vi "LINC Read Command.vi"(8 "error in (no error)":errorcluster, 9 "Options":T1, 10 "start field (default)":i32=-1, 11 "LINC session":refnum<class "LINC.lvclass">) -> (0 "error out":errorcluster, 1 "cmd data":string, 2 "cmd name":string, 3 "dup LINC session":refnum<class "LINC.lvclass">, 4 "application command":bool, 5 "GUID":string, 6 "cmd text":string, 7 "cmd origin":T2)   [LabVIEW 2018, in "STEPkgDriver_LINC.lvlib" / "LINC.lvclass"]
uses:
  LINC.lvclass
  STEPkgDriver_LINC.lvlib
  LINC Global Mode.ctl
  LINC Command Origin.ctl
  LINC Read Command Options.ctl
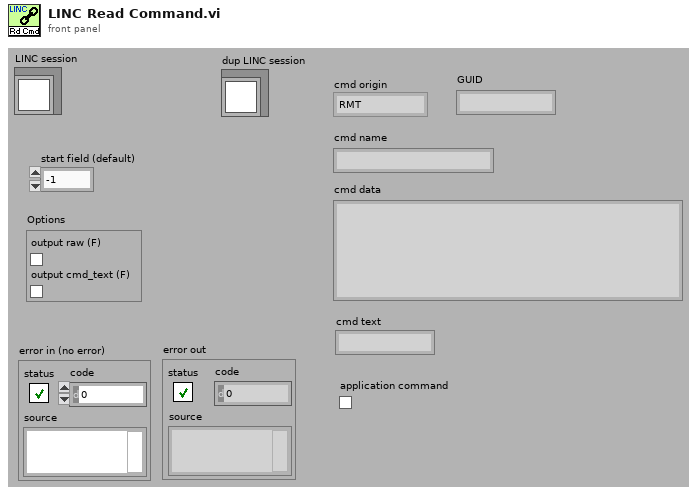
[diagram p1: front panel]
types:
  T1 = typedef "STEPkgDriver_LINC.lvlib/LINC Read Command Options.ctl" = cluster{"output raw (F)":bool, "output cmd_text (F)":bool}
  T2 = typedef "STEPkgDriver_LINC.lvlib/LINC Command Origin.ctl" = enum8{"RMT", "LCL"}
  T3 = typedef "STEPkgDriver_LINC.lvlib/LINC Global Mode.ctl" = enum16{"INIT", "CLEAR", "ADD_PKT_HDR", "ADD_PKT", "GET_PKT_NAMES", "GET_PKT_DESC", "GET_PKT_HDR", "GET_PKT", "SET_PKT", "SET_DATA", "SIM_EN", "SIM_DS"}
  T4 = typedef "STEPkgDriver_LINC.lvlib/LINC Format Prototype.ctl" = cluster{"type":string, "bit offset":i32, "bit size":i32, "format":string, "unit":string, "description":string, "state values":i64[], "states":string[], "max":string, "min":string, "default":string, "array":bool, "bit element size":i32, "poly bound":dbl[], "poly scale":cluster{"coefficients":dbl[]}[], "labview size":i32, "simulate":bool, "ID":bool, "required":bool}
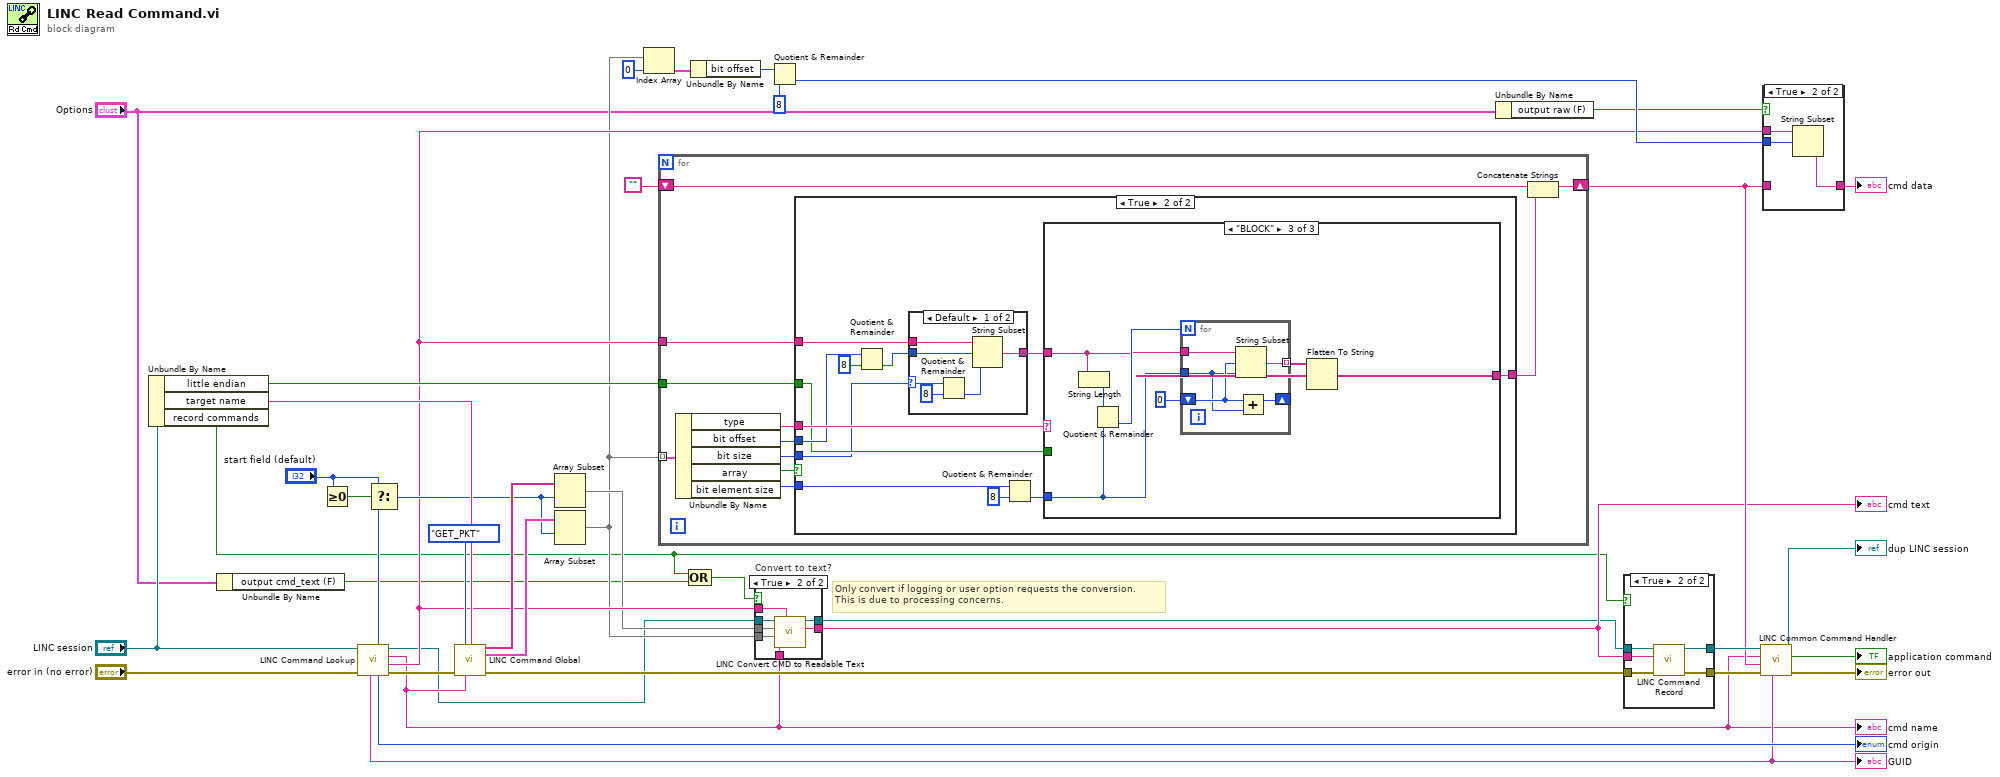
[diagram p0: block diagram]
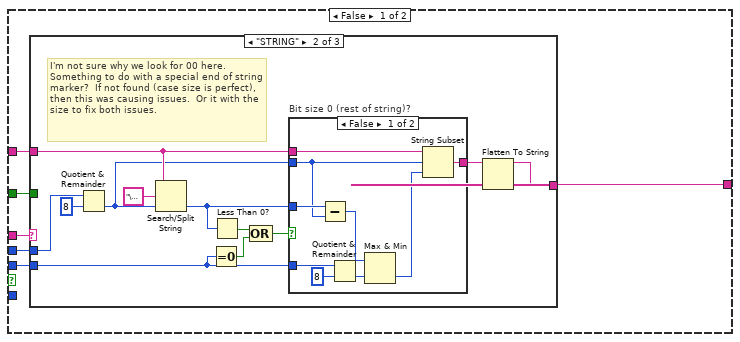
[diagram p3: hidden frame]
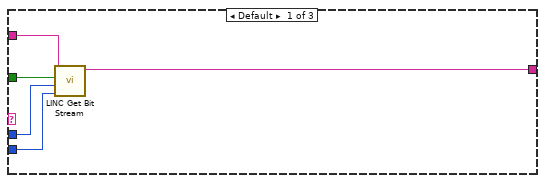
[diagram p4: hidden frame]
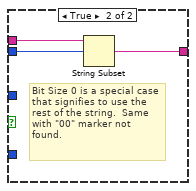
[diagram p5: hidden frame]
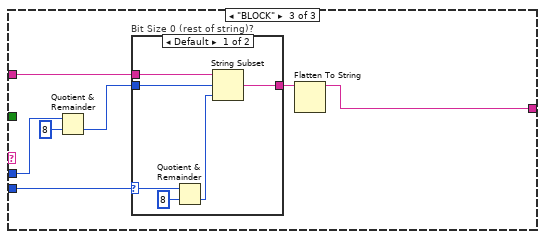
[diagram p6: hidden frame]
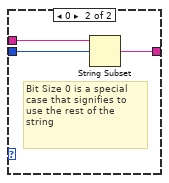
[diagram p7: hidden frame]
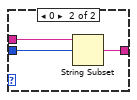
[diagram p8: hidden frame]
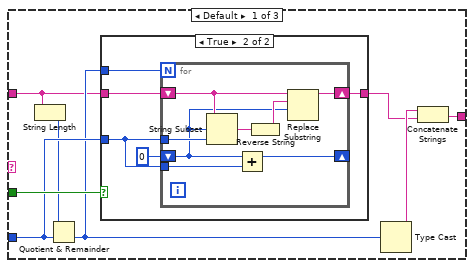
[diagram p9: hidden frame]
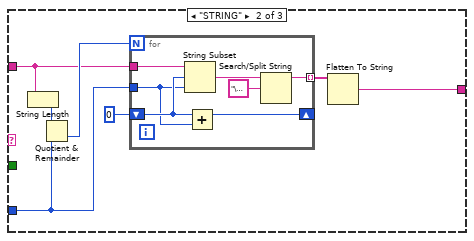
[diagram p11: hidden frame]
diagram:
  # "Only convert if logging or user option requests the conversion.\nThis is due to processing concerns."
  n1 = Unbundle By Name("LINC session") -> ("little endian"=w29:bool, "target name"=w32:string, "record commands"=w3:bool)
  n2 = Unbundle By Name("Options") -> ("output cmd_text (F)"=w2:bool)
  n3 = Greater Or Equal To 0?(x="start field (default)") -> (x >= 0?=w28:bool)
  n4 = call "LINC Command Lookup.vi"("error in (no error)"="error in (no error)", "LINC session"="LINC session") -> ("error out"=w31:errorcluster, "cmd data"=w13:string, "cmd name"=w12:string, "dup LINC session"=w8:refnum<class "LINC.lvclass">, "cmd origin"=→"cmd origin":T2, "cmd header fields"=w27:i32, "cmd GUID"=w14:string)  [unwired: 3 in]
  "cmd name" <- w12
  "GUID" <- w14
  n5 = Select(t="start field (default)", s=w28, f=w27) -> (s? t:f=w16:i32)
  n6 = call "LINC Command Global.vi"("mode"=LINC_Global_Mode."GET_PKT", "target name"=w32, "error in (no error)"=w31, "packet name"=w12) -> ("values out"=w18:string[], "item formats out"=w17:T4[], "error out"=w36:errorcluster)  [unwired: 7 in, 2 out]
  n7 = Array Subset(array=w18, index=w16) -> (w11:string[])  [unwired: 1 in]
  n8 = Array Subset(array=w17, index=w16) -> (w10:T4[])  [unwired: 1 in]
  n9 = Index Array(array=w10, index=0) -> (element=w23:T4)
  n10 = for {
    shift-right: [w51] -> w19
    shift-left: "" -> [w45]
    tunnel: w13 -> [w46]
    tunnel: w29 -> [w42]
    tunnel: w10 -> [w41] mode=indexing
    n11 = Unbundle By Name(w41) -> ("type"=w47:string, "bit offset"=w43:i32, "bit size"=w50:i32, "array"=w48:bool, "bit element size"=w49:i32)
    n12 = case shown="True" w48 {
      tunnel: w47 -> [w57 w113]
      tunnel: w50 -> [w55 w103]
      tunnel: [w56 w114] -> w44
      tunnel: w49 -> [_ w110]
      tunnel: w43 -> [w53 w106]
      tunnel: w46 -> [w54 w107]
      tunnel: w42 -> [w52 w104]
      frame False {
        n13 = case shown="\"STRING\"" w57 {
          tunnel: w55 -> [w60 w64 w87]
          tunnel: [w59 w69 w89] -> w56
          tunnel: w54 -> [w62 w71 w91]
          tunnel: w53 -> [w61 w72 w92]
          tunnel: w52 -> [w58 _ _]
          frame Default {
            n14 = call "LINC Get Bit Stream.vi"("bit size"=w60, "bit offset"=w61, "little endian"=w58, "data in"=w62) -> ("data out"=w59:string)  [unwired: 6 in, 1 out]
          }
          frame "STRING" {
            # "I'm not sure why we look for 00 here. Something to do with a special end of string marker?  If not found (case size is perfect), then this was causing issues.  Or it with the size to fix both issues."
            n15 = Quotient & Remainder(x=w72, y=8) -> (floor(x/y)=w70:i32)  [unwired: 1 out]
            n16 = Search/Split String(string=w71, search string/char (-)="\u0000", offset (0)=w70) -> (offset of match=w67:i32)  [unwired: 2 out]
            n17 = Equal To 0?(x=w64) -> (x = 0?=w65:bool)
            n18 = Less Than 0?(x=w67) -> (x < 0?=w66:bool)
            n19 = Compound Arithmetic op=OR(w66, w65) -> (w63:bool)
            n20 = case "Bit size 0 (rest of string)?" shown="False" w63 {
              tunnel: w71 -> [w83 w86]
              tunnel: w67 -> [w82 _]
              tunnel: w70 -> [w81 w85]
              tunnel: [w76 w84] -> w68
              tunnel: w64 -> [w75 _]
              frame False {
                n21 = Subtract(x=w82, y=w81) -> (x-y=w79:i32)
                n22 = Quotient & Remainder(x=w75, y=8) -> (floor(x/y)=w78:i32)  [unwired: 1 out]
                n23 = Max & Min(x=w79, y=w78) -> (min(x,y)=w77:i32)  [unwired: 1 out]
                n24 = String Subset(string=w83, offset (0)=w81, length (rest)=w77) -> (substring=w76:string)
              }
              frame True {
                # "Bit Size 0 is a special case that signifies to use the rest of the string.  Same with \"00\" marker not found."
                n25 = String Subset(string=w86, offset (0)=w85) -> (substring=w84:string)  [unwired: 1 in]
              }
            }
            n26 = Flatten To String(anything=w68) -> (data string=w69:string)  [unwired: 3 in, 2 out]
          }
          frame "BLOCK" {
            n27 = Quotient & Remainder(x=w92, y=8) -> (floor(x/y)=w90:i32)  [unwired: 1 out]
            n28 = case "Bit Size 0 (rest of string)?" shown="Default" w87 {
              selector: w87 -> [w94 _]
              tunnel: w91 -> [w99 w102]
              tunnel: w90 -> [w98 w100]
              tunnel: [w97 w101] -> w88
              frame Default {
                n29 = Quotient & Remainder(x=w94, y=8) -> (floor(x/y)=w96:i32)  [unwired: 1 out]
                n30 = String Subset(string=w99, offset (0)=w98, length (rest)=w96) -> (substring=w97:string)
              }
              frame 0 {
                # "Bit Size 0 is a special case that signifies to use the rest of the string"
                n31 = String Subset(string=w102, offset (0)=w100) -> (substring=w101:string)  [unwired: 1 in]
              }
            }
            n32 = Flatten To String(anything=w88) -> (data string=w89:string)  [unwired: 3 in, 2 out]
          }
        }
      }
      frame True {
        n33 = Quotient & Remainder(x=w106, y=8) -> (floor(x/y)=w109:i32)  [unwired: 1 out]
        n34 = case shown="Default" w103 {
          selector: w103 -> [w115 _]
          tunnel: w109 -> [w120 w123]
          tunnel: w107 -> [w118 w122]
          tunnel: [w117 w121] -> w105
          frame Default {
            n35 = Quotient & Remainder(x=w115, y=8) -> (floor(x/y)=w116:i32)  [unwired: 1 out]
            n36 = String Subset(string=w118, offset (0)=w120, length (rest)=w116) -> (substring=w117:string)
          }
          frame 0 {
            n37 = String Subset(string=w122, offset (0)=w123) -> (substring=w121:string)  [unwired: 1 in]
          }
        }
        n38 = Quotient & Remainder(x=w110, y=8) -> (floor(x/y)=w111:i32)  [unwired: 1 out]
        n39 = case shown="\"BLOCK\"" w113 {
          tunnel: [w130 w148 w162] -> w114
          tunnel: w111 -> [w127 w150 w164]
          tunnel: w105 -> [w125 w147 w161]
          tunnel: w104 -> [w128 _ _]
          frame Default {
            n40 = String Length(string=w125) -> (length=w124:i32)
            n41 = Quotient & Remainder(x=w124, y=w127) -> (floor(x/y)=w126:i32)  [unwired: 1 out]
            n42 = case shown="True" w128 {
              tunnel: w125 -> [w132 w136]
              tunnel: [w132 w135] -> w129
              tunnel: w127 -> [_ w134]
              tunnel: w126 -> [_ w133]
              frame False {
              }
              frame True {
                n43 = for {
                  N: w133 -> [_]
                  shift-right: [w140] -> w135
                  shift-left: w136 -> [w141]
                  shift-right: [w144] -> _
                  shift-left: 0 -> [w138]
                  tunnel: w134 -> [w145]
                  tunnel: w134 -> [w143]
                  n44 = String Subset(string=w141, offset (0)=w138, length (rest)=w145) -> (substring=w142:string)
                  n45 = Add(x=w138, y=w143) -> (x+y=w144:i32)
                  n46 = Reverse String(1:w142) -> (0:w139:string)
                  n47 = Replace Substring(3:w138, 4:w139, 5:w141) -> (1:w140:string)  [unwired: 1 in, 1 out]
                }
              }
            }
            n48 = Type Cast(x=w126) -> (*(type *) &x=w131:string)  [unwired: 1 in]
            n49 = Concatenate Strings(w131, w129) -> (w130:string)
          }
          frame "STRING" {
            n50 = String Length(string=w147) -> (length=w146:i32)
            n51 = Quotient & Remainder(x=w146, y=w150) -> (floor(x/y)=w151:i32)  [unwired: 1 out]
            n52 = for {
              N: w151 -> [_]
              tunnel: w150 -> [w156]
              tunnel: w147 -> [w159]
              shift-right: [w157] -> _
              shift-left: 0 -> [w158]
              tunnel: [w153] -> w149 mode=indexing
              n53 = String Subset(string=w159, offset (0)=w158, length (rest)=w156) -> (substring=w154:string)
              n54 = Add(x=w158, y=w156) -> (x+y=w157:i32)
              n55 = Search/Split String(string=w154, search string/char (-)="\u0000") -> (substring before match=w153:string)  [unwired: 3 out]
            }
            n56 = Flatten To String(anything=w149) -> (data string=w148:string)  [unwired: 3 in, 2 out]
          }
          frame "BLOCK" {
            n57 = String Length(string=w161) -> (length=w160:i32)
            n58 = Quotient & Remainder(x=w160, y=w164) -> (floor(x/y)=w165:i32)  [unwired: 1 out]
            n59 = for {
              N: w165 -> [_]
              tunnel: w164 -> [w168]
              tunnel: w161 -> [w171]
              shift-right: [w169] -> _
              shift-left: 0 -> [w170]
              tunnel: [w167] -> w163 mode=indexing
              n60 = String Subset(string=w171, offset (0)=w170, length (rest)=w168) -> (substring=w167:string)
              n61 = Add(x=w170, y=w168) -> (x+y=w169:i32)
            }
            n62 = Flatten To String(anything=w163) -> (data string=w162:string)  [unwired: 3 in, 2 out]
          }
        }
      }
    }
    n63 = Concatenate Strings(w45, w44) -> (w51:string)
  }
  n64 = Compound Arithmetic op=OR(w3, w2) -> (w1:bool)
  n65 = Unbundle By Name(w23) -> ("bit offset"=w22:i32)
  n66 = case "Convert to text?" shown="True" w1 {
    tunnel: w13 -> [_ w179]
    tunnel: w12 -> [_ w178]
    tunnel: w11 -> [_ w177]
    tunnel: w10 -> [_ w176]
    tunnel: [_ w175] -> w9
    tunnel: w8 -> [w172 w174]
    tunnel: [w172 w173] -> w6
    frame False {
    }
    frame True {
      n67 = call "LINC Convert CMD to Readable Text.vi"("command name in"=w178, "command data in"=w179, "parameter formats"=w176, "parameter names"=w177, "LINC in"=w174) -> ("Cmd Text"=w175:string, "LINC out"=w173:refnum<class "LINC.lvclass">)  [unwired: 5 in]
    }
  }
  "cmd text" <- w9
  n68 = Quotient & Remainder(x=w22, y=8) -> (floor(x/y)=w20:i32)  [unwired: 1 out]
  n69 = Unbundle By Name("Options") -> ("output raw (F)"=w5:bool)
  n70 = case shown="True" w3 {
    tunnel: [w180 w186] -> w37
    tunnel: w36 -> [w180 w185]
    tunnel: [w181 w184] -> w35
    tunnel: w6 -> [w181 w183]
    tunnel: w9 -> [_ w182]
    frame False {
    }
    frame True {
      n71 = call "LINC Command Record.vi"("error in (no error)"=w185, "command text"=w182, "LINC session"=w183) -> ("error out"=w186:errorcluster, "dup LINC session"=w184:refnum<class "LINC.lvclass">)  [unwired: 7 in]
    }
  }
  n72 = call "LINC Common Command Handler.vi"("GUID"=w14, "error in (no error)"=w37, "command data in"=w19, "command name in"=w12, "LINC session"=w35) -> ("error out"=→"error out":errorcluster, "application command"=→"application command":bool, "dup LINC session"=→"dup LINC session":refnum<class "LINC.lvclass">)  [unwired: 4 in]
  n73 = case shown="True" w5 {
    tunnel: w13 -> [_ w190]
    tunnel: [w187 w189] -> w24
    tunnel: w20 -> [_ w188]
    tunnel: w19 -> [w187 _]
    frame False {
    }
    frame True {
      n74 = String Subset(string=w190, offset (0)=w188) -> (substring=w189:string)  [unwired: 1 in]
    }
  }
  "cmd data" <- w24
